vi "Temp Variables.vi"() -> ()   [LabVIEW 2015]
uses:
  <vilib>/Rock Robotics/WPI/CAN/TalonSRX/WPI_CANTalonSRX_APIControlMode.ctl
  Subsystem VIs/Drive SS/Drive Subsystem State.ctl
panel:
  out "Robot AutoTargeting":bool
  out "Robot Trying to Turn To heading":bool
  out "Robot acquired target Lock":bool
  out "Robot Recently Run Auto":bool
  out "Robot is Shooter Forward?":bool
  out "Defense Drive Mode":bool
  out "In Test Mode":bool
  out "Attempting to Cock":bool
  out "Robot in Positional Control":bool
  in  "Drive/Climb State":T1
  in  "Drive Talon Mode":T2=enum."Speed"
  out "Temp Hold":bool
  out "Robot has been disabled":bool
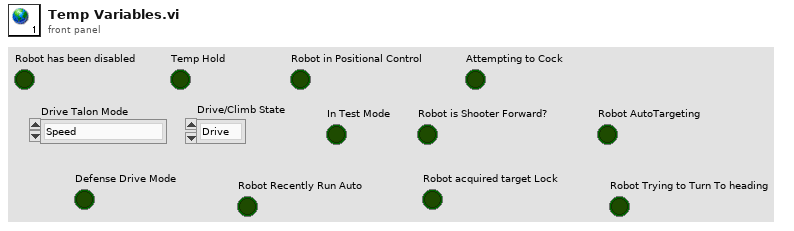
[diagram p1: front panel]
types:
  T1 = typedef "Drive Subsystem State.ctl" = enum16{"Drive", "Climb", "Auto Target"}
  T2 = typedef "WPI_CANTalonSRX_APIControlMode.ctl" = enum8{"Percent VBus", "Speed", "Position", "Slave", "Unchanged / Invalid", "Voltage Compensation", "Current", "Motion Profile"}
diagram:
